vi "viewerUpdateDataVectors.vi"(8 "viewerDataVectors":T2, 10 "Cluster":T1, 11 "viewer.lvclass":refnum<class "viewer.lvclass">) -> (0 "viewerDataVectorsOut":T2, 3 "viewer.lvclassOut":refnum<class "viewer.lvclass">)   [LabVIEW 2011, in "viewer.lvclass"]
uses:
  Pollers/ttm_poller_panel_class/viewer.lvclass
  viewerDataVectors.ctl
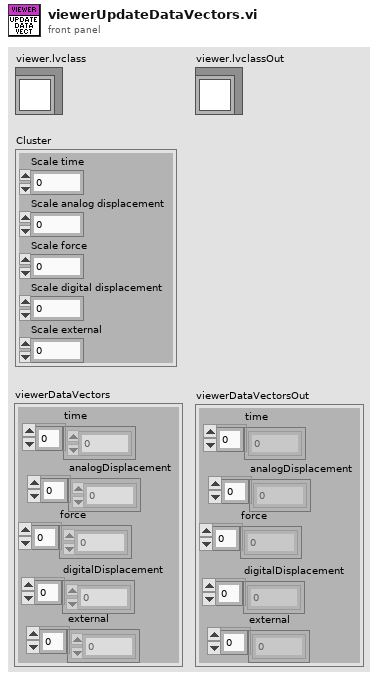
[diagram p1: front panel]
types:
  T1 = cluster{"Scale time":dbl, "Scale analog displacement":dbl, "Scale force":dbl, "Scale digital displacement":dbl, "Scale external":dbl}
  T2 = typedef "viewer.lvclass/viewerDataVectors.ctl" = cluster{"time":dbl[], "analogDisplacement":dbl[], "external":dbl[], "force":dbl[], "digitalDisplacement":dbl[]}
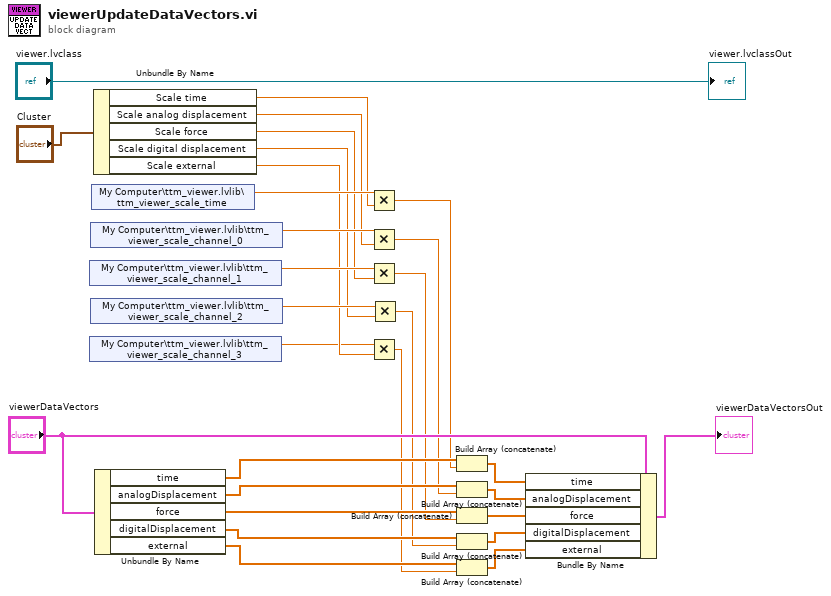
[diagram p0: block diagram]
diagram:
  n1 = shared-variable "My Computer\\ttm_viewer.lvlib\\ttm_viewer_scale_channel_1"() -> (w10:dbl)  [unwired: 1 in, 1 out]
  n2 = shared-variable "My Computer\\ttm_viewer.lvlib\\ttm_viewer_scale_channel_3"() -> (w3:dbl)  [unwired: 1 in, 1 out]
  n3 = shared-variable "My Computer\\ttm_viewer.lvlib\\ttm_viewer_scale_channel_0"() -> (w13:dbl)  [unwired: 1 in, 1 out]
  n4 = shared-variable "My Computer\\ttm_viewer.lvlib\\ttm_viewer_scale_channel_2"() -> (w7:dbl)  [unwired: 1 in, 1 out]
  n5 = shared-variable "My Computer\\ttm_viewer.lvlib\\ttm_viewer_scale_time"() -> (w16:dbl)  [unwired: 1 in, 1 out]
  n6 = Unbundle By Name("Cluster") -> ("Scale time"=w15:dbl, "Scale analog displacement"=w12:dbl, "Scale force"=w9:dbl, "Scale digital displacement"=w5:dbl, "Scale external"=w4:dbl)
  n7 = Unbundle By Name("viewerDataVectors") -> ("time"=w18:dbl[], "analogDisplacement"=w26:dbl[], "force"=w24:dbl[], "digitalDisplacement"=w22:dbl[], "external"=w20:dbl[])
  n8 = Multiply(x=w16, y=w15) -> (x*y=w14:dbl)
  n9 = Multiply(x=w13, y=w12) -> (x*y=w11:dbl)
  n10 = Multiply(x=w10, y=w9) -> (x*y=w8:dbl)
  n11 = Multiply(x=w3, y=w4) -> (x*y=w2:dbl)
  n12 = Multiply(x=w7, y=w5) -> (x*y=w6:dbl)
  n13 = Build Array (concatenate)(w18, w14) -> (w27:dbl[])
  n14 = Build Array (concatenate)(w26, w11) -> (w25:dbl[])
  n15 = Build Array (concatenate)(w24, w8) -> (w23:dbl[])
  n16 = Build Array (concatenate)(w22, w6) -> (w21:dbl[])
  n17 = Build Array (concatenate)(w20, w2) -> (w19:dbl[])
  n18 = Bundle By Name(cluster="viewerDataVectors", "time"=w27, "analogDisplacement"=w25, "force"=w23, "digitalDisplacement"=w21, "external"=w19) -> (→"viewerDataVectorsOut":T2)
  "viewer.lvclassOut" <- "viewer.lvclass"
